vi "DCPower_TurnOff_KeepReference.vi"(2 "error in (no error)":errorcluster, 3 "DCPower_byInstrument_input":T1(array[cluster])) -> (0 "error out":errorcluster, 1 "DCPower_byInstrument_output":T1(array[cluster]))   [LabVIEW 2019]
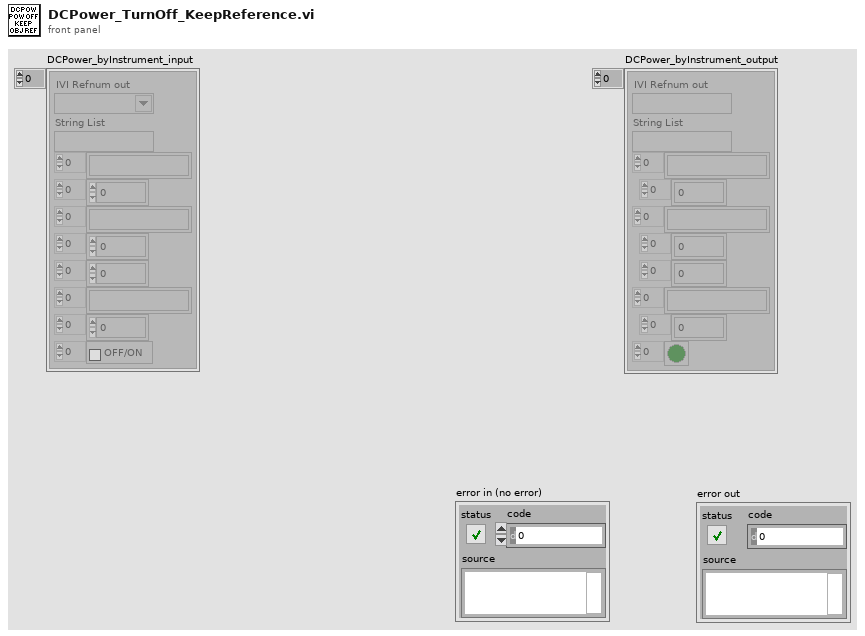
[diagram p1: front panel]
types:
  T1 = cluster{"IVI Refnum out":refnum<k15>, "String List":string, string[], dbl[], string[], dbl[], dbl[], string[], dbl[], bool[]}[]
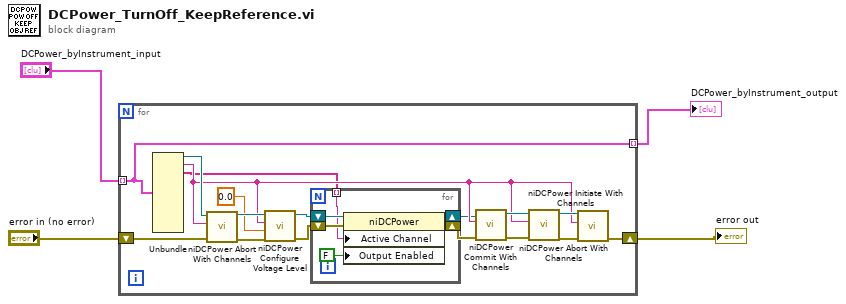
[diagram p0: block diagram]
diagram:
  n1 = for {
    tunnel: "DCPower_byInstrument_input" -> [w10] mode=indexing
    shift-right: [w11] -> w3
    shift-left: "error in (no error)" -> [w18]
    tunnel: [w10] -> w2 mode=indexing
    n2 = Unbundle(w10) -> ("IVI Refnum out"=w19:refnum<k15>, "String List"=w12:string, w5:string[])  [unwired: 7 out]
    n3 = call <instrlib>:"niDCPower Abort With Channels.vi"("error in (no error)"=w18, "channel name"=w12, "instrument handle"=w19) -> ("error out"=w21:errorcluster, "instrument handle out"=w20:refnum<k15>)  [unwired: 7 in]
    n4 = call <instrlib>:"niDCPower Configure Voltage Level.vi"("error in (no error)"=w21, "voltage level"=0.0, "channel name"=w12, "instrument handle"=w20) -> ("error out"=w9:errorcluster, "instrument handle out"=w8:refnum<k15>)  [unwired: 6 in]
    n5 = for {
      shift-right: [w24] -> w6
      shift-left: w9 -> [w27]
      shift-right: [w25] -> w7
      shift-left: w8 -> [w26]
      tunnel: w5 -> [w22] mode=indexing
      n6 = property class="niDCPower"(reference=w26, error in=w27, "Active Channel"=w22, "Output Enabled"=FALSE ("Source:Output Enabled")) -> (reference out=w25:refnum<k15>, error out=w24:errorcluster)
    }
    n7 = call <instrlib>:"niDCPower Commit With Channels.vi"("error in (no error)"=w6, "channel name"=w12, "instrument handle"=w7) -> ("error out"=w15:errorcluster, "instrument handle out"=w16:refnum<k15>)  [unwired: 7 in]
    n8 = call <instrlib>:"niDCPower Initiate With Channels.vi"("error in (no error)"=w15, "channel name"=w12, "instrument handle"=w16) -> ("error out"=w14:errorcluster, "instrument handle out"=w13:refnum<k15>)  [unwired: 7 in]
    n9 = call <instrlib>:"niDCPower Abort With Channels.vi"("error in (no error)"=w14, "channel name"=w12, "instrument handle"=w13) -> ("error out"=w11:errorcluster)  [unwired: 7 in, 1 out]
  }
  "error out" <- w3
  "DCPower_byInstrument_output" <- w2
